vi "Move Methods.vi"() -> ()   [LabVIEW 2018]
panel:
  out "Array":errorcluster[](array[cluster])
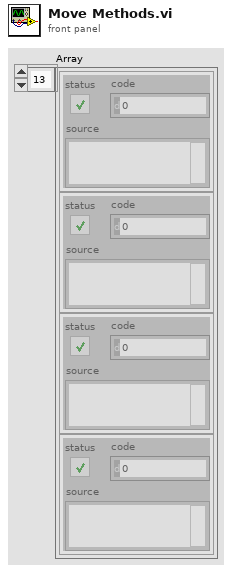
[diagram p1: front panel]
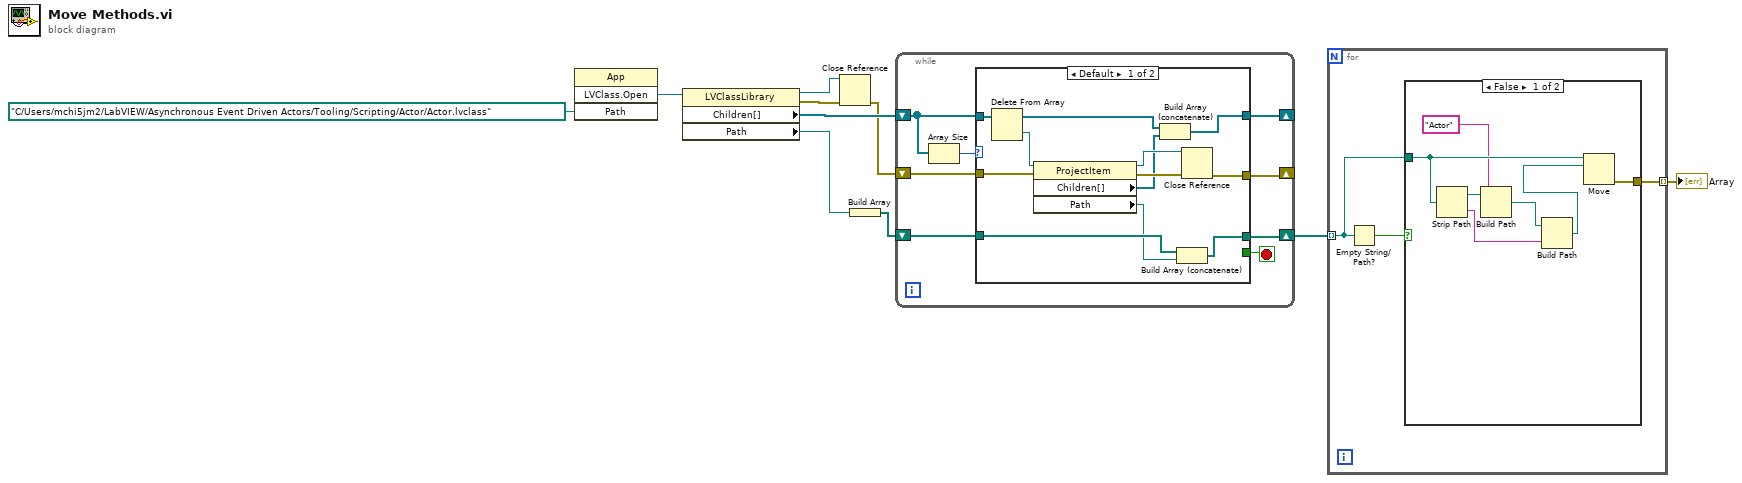
[diagram p0: block diagram]
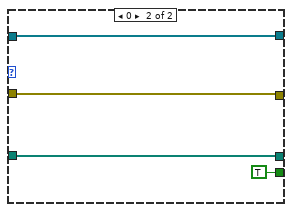
[diagram p3: hidden frame]
diagram:
  n1 = invoke class="App" method="LVClass.Open"("Path"=path "C:/Users/mchi5jm2/LabVIEW/Asynchronous Event Driven Actors/Tooling/Scripting/Actor/Actor.lvclass") -> ("LVClass.Open"=w9:refnum<vi>)  [unwired: 3 in, 3 out]
  n2 = property class="LVClassLibrary"(reference=w9) -> (reference out=w6:refnum<vi>, error out=w7:errorcluster, "Children[]"=w8:refnum<vi>[], "Path"=w3:path)  [unwired: 1 in]
  n3 = Close Reference(reference=w6, error in (no error)=w7) -> (error out=w5:errorcluster)
  n4 = Build Array(w3) -> (w4:path[])
  n5 = while {
    shift-right: [w13] -> _
    shift-left: w5 -> [w15]
    shift-right: [w11] -> _
    shift-left: w8 -> [w16]
    shift-right: [w12] -> w2
    shift-left: w4 -> [w14]
    stop <- w17 stop-if-true
    n6 = Array Size(array=w16) -> (size(s)=w18:i32)
    n7 = case shown="Default" w18 {
      tunnel: [_ TRUE] -> w17
      tunnel: w16 -> [w30 w31]
      tunnel: w15 -> [w27 w33]
      tunnel: w14 -> [w23 w32]
      tunnel: [w24 w33] -> w13
      tunnel: [w22 w32] -> w12
      tunnel: [w21 w31] -> w11
      frame Default {
        n8 = Delete From Array(array=w30) -> (deleted portion=w29:refnum<vi>, array with subset deleted=w28:refnum<vi>[])  [unwired: 2 in]
        n9 = property class="ProjectItem"(reference=w29, error in=w27) -> (reference out=w25:refnum<vi>, error out=w26:errorcluster, "Children[]"=w19:refnum<vi>[], "Path"=w20:path)
        n10 = Build Array (concatenate)(w28, w19) -> (w21:refnum<vi>[])
        n11 = Build Array (concatenate)(w23, w20) -> (w22:path[])
        n12 = Close Reference(reference=w25, error in (no error)=w26) -> (error out=w24:errorcluster)
      }
      frame 0 {
      }
    }
  }
  n13 = for {
    tunnel: w2 -> [w36] mode=indexing
    tunnel: [w35] -> w1 mode=indexing
    n14 = Empty String/Path?(string/path=w36) -> (empty?=w37:bool)
    n15 = case shown="False" w37 {
      tunnel: w36 -> [w44 _]
      tunnel: [w38 _] -> w35
      frame False {
        n16 = Strip Path(path=w44) -> (stripped path=w43:path, name=w41:string)
        n17 = Build Path(base path=w43, name or relative path="Actor") -> (appended path=w42:path)
        n18 = Build Path(base path=w42, name or relative path=w41) -> (appended path=w39:path)
        n19 = Move(source path=w44, 10:w39) -> (error out=w38:errorcluster)  [unwired: 3 in, 2 out]
      }
      frame True {
      }
    }
  }
  "Array" <- w1
